vi "vel_cal_Reference.vi"(8 "error in (no error)":errorcluster caption="错误输入（无错误）", 10 "值(信号)":cluster{"rot_z":dbl, "lin_x":dbl}, 11 "Map输入":refnum<class "Map.lvclass">) -> (0 "error out":errorcluster caption="错误输出", 3 "Map输出":refnum<class "Map.lvclass">)   [LabVIEW 2014, in "Map.lvlib" / "Map.lvclass"]
uses:
  Map.lvclass
  Map.lvclass/Map.ctl
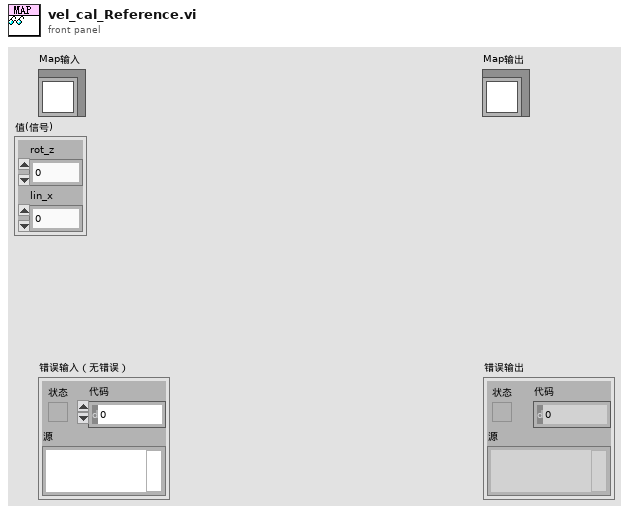
[diagram p1: front panel]
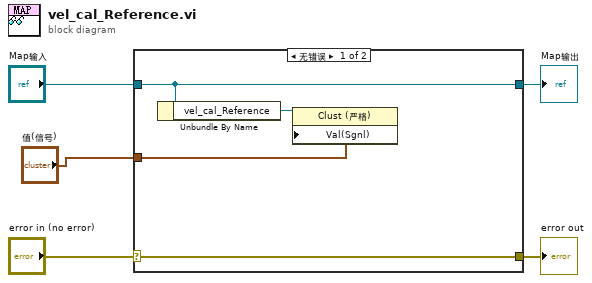
[diagram p0: block diagram]
diagram:
  n1 = case shown="无错误" "error in (no error)" {
    selector: "error in (no error)" -> [w9 w10]
    tunnel: [w9 w10] -> w4
    tunnel: [w8 w11] -> w2
    tunnel: "Map输入" -> [w8 w11]
    tunnel: "值(信号)" -> [w6 _]
    frame No Error {
      n2 = Unbundle By Name(w8) -> ("vel_cal_Reference"=w7:refnum<vi>)
      n3 = property class="Clust (严格)"(reference=w7, "Val(Sgnl)"=w6) -> ()  [unwired: 1 in, 2 out]
    }
    frame Error {
    }
  }
  "error out" <- w4
  "Map输出" <- w2
